vi "Write Frequency.vi"(8 "error in":errorcluster, 10 "frequency":T1, 11 "PWM output channel in":refnum<class "PWM Output Channel.lvclass">) -> (0 "error out":errorcluster, 3 "PWM output channel out":refnum<class "PWM Output Channel.lvclass">)   [LabVIEW 2020, in "Scan Engine Scripting.lvlib" / "PWM Output Channel.lvclass"]
uses:
  PWM Output Channel.lvclass
  Frequency.ctl
  PWM Output Channel.lvclass/PWM Output Channel.ctl
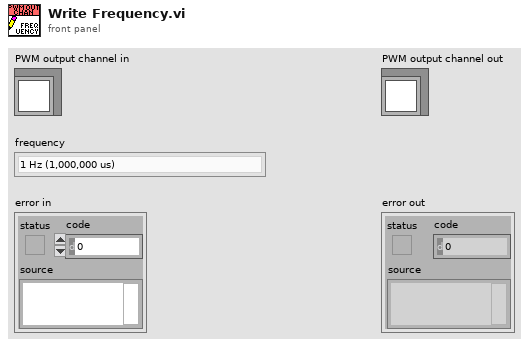
[diagram p1: front panel]
types:
  T1 = typedef "Scan Engine Scripting.lvlib/PWM Output Channel.lvclass/Frequency.ctl" = enum16{"1 Hz (1,000,000 us)", "50 Hz (20,000 us)", "250 Hz (4,000 us)", "500 Hz (2,000 us)", "1 kHz (1,000 us)", "5 kHz (200 us)", "10 kHz (100 us)", "20 kHz (50 us)"}
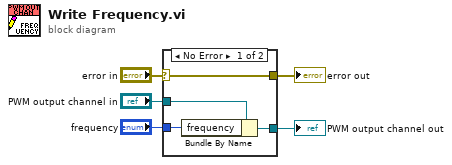
[diagram p0: block diagram]
diagram:
  n1 = case shown="No Error" "error in" {
    selector: "error in" -> [w9 w10]
    tunnel: [w9 w10] -> w4
    tunnel: [w7 w11] -> w2
    tunnel: "PWM output channel in" -> [w8 w11]
    tunnel: "frequency" -> [w6 _]
    frame No Error {
      n2 = Bundle By Name(cluster=w8, "frequency"=w6) -> (w7:refnum<class "PWM Output Channel.lvclass">)
    }
    frame Error {
    }
  }
  "error out" <- w4
  "PWM output channel out" <- w2
